vi "testStatusView.vi"(10 "UserEvents in":refnum<class "UserEvents.lvclass">) -> ()   [LabVIEW 2013, in "M2AADTViews.lvlib"]
uses:
  UserEvents/UserEvents.lvclass
  UserEvents/UserEvents.lvclass/UserEvents.ctl
  Typedefs/StateSelector.ctl
  M2AADTViews.lvlib
  Typedefs/M2AADTTypedefs.lvlib
panel:
  out "Demanded Steps":u32 caption="of"
  out "Demanded Cycles":u32 caption="of"
  out "Log Path":path
  out "Active Profile Step":u32
  out "Active Cycle":u32
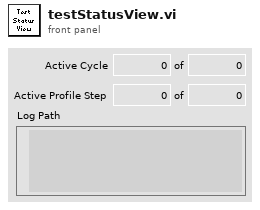
[diagram p1: front panel]
types:
  T1 = typedef "M2AADTTypedefs.lvlib/PubDataEvents.ctl" = cluster{"State":refnum<user-event>, "ErrorCode":refnum<user-event>, "OutputData":refnum<user-event>, "InputData":refnum<user-event>, "ControllerData":refnum<user-event>, "TestStatus":refnum<user-event>, "LogPath":refnum<user-event>, "StiffnessData":refnum<user-event>}
  T2 = cluster{"Event Registration Refnum":refnum<event-registration>, "Event Registration Refnum":refnum<event-registration>, "Event Registration Refnum":refnum<event-registration>}
  T3 = typedef "M2AADTTypedefs.lvlib/StateSelector.ctl" = enum16{"EndingCycleState", "FaultState", "InteractiveMotionState", "MovingToNewForceState", "OffState", "PausingState", "StandbyState", "StoppedState"}
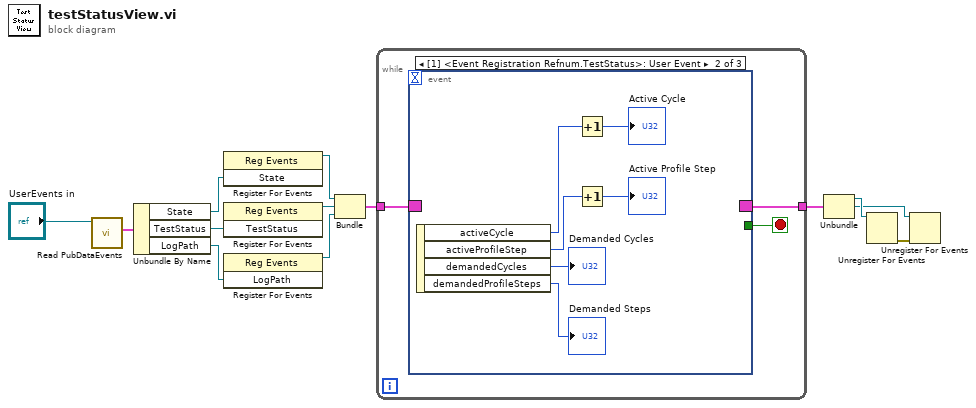
[diagram p0: block diagram]
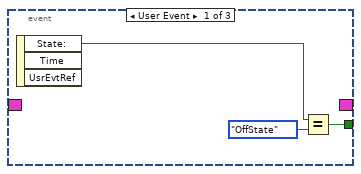
[diagram p2: hidden frame]
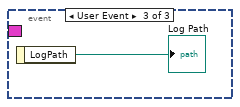
[diagram p3: hidden frame]
diagram:
  n1 = call "Read PubDataEvents.vi"("UserEvents in"="UserEvents in") -> ("PubDataEvents"=w9:T1)  [unwired: 9 in, 1 out]
  n2 = Unbundle By Name(w9) -> ("State"=w10:refnum<user-event>, "TestStatus"=w12:refnum<user-event>, "LogPath"=w2:refnum<user-event>)
  n3 = register-events(w10) -> (reference out=w11:refnum<event-registration>)  [unwired: 2 in, 1 out]
  n4 = register-events(w12) -> (reference out=w13:refnum<event-registration>)  [unwired: 2 in, 1 out]
  n5 = register-events(w2) -> (reference out=w1:refnum<event-registration>)  [unwired: 2 in, 1 out]
  n6 = Bundle("Event Registration Refnum"=w11, "Event Registration Refnum"=w13, "Event Registration Refnum"=w1) -> (w8:T2)  [unwired: 1 in]
  n7 = while {
    tunnel: w8 -> [w16]
    tunnel: [w15] -> w7
    stop <- w14 stop-if-true
    n8 = event shown="[1] <Event Registration Refnum.TestStatus>: User Event" {
      selector: w16 -> [_ _ _]
      dyn-events: [_ _ _] -> w15
      timeout: _ -> [_ _ _]
      tunnel: [w17 _ _] -> w14
      event User Event {
        n9 = event-data() -> ("State:"=w18:T3)  [unwired: 1 in, 2 out]
        n10 = Equal?(x=w18, y=StateSelector."OffState") -> (x = y?=w17:bool)
      }
      event User Event {
        n11 = event-data() -> ("activeCycle"=w25:u32, "activeProfileStep"=w24:u32, "demandedCycles"=→"Demanded Cycles":u32, "demandedProfileSteps"=→"Demanded Steps":u32)  [unwired: 1 in]
        n12 = Increment(x=w25) -> (x+1=→"Active Cycle":u32)
        n13 = Increment(x=w24) -> (x+1=→"Active Profile Step":u32)
      }
      event User Event {
        n14 = event-data() -> ("LogPath"=→"Log Path":path)  [unwired: 1 in]
      }
    }
  }
  n15 = Unbundle(w7) -> ("Event Registration Refnum"=w6:refnum<event-registration>, "Event Registration Refnum"=w4:refnum<event-registration>)  [unwired: 1 out]
  n16 = Unregister For Events(event registration refnum=w6) -> (error out=w5:errorcluster)  [unwired: 1 in]
  n17 = Unregister For Events(event registration refnum=w4, error in=w5) -> ()  [unwired: 1 out]
